vi "Decrypt Play Action.vi"(1 "Encrypted Play Action":string, 2 "Opponent's Move":T1) -> (0 "My Move":T1)   [LabVIEW 2020, in "AoC 2022.lvlib"]
uses:
  AoC 2022.lvlib
  Play Item.ctl
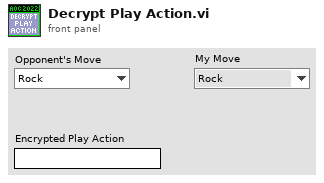
[diagram p1: front panel]
types:
  T1 = typedef "AoC 2022.lvlib/Play Item.ctl" = enum16{"Rock", "Paper", "Scissor"}
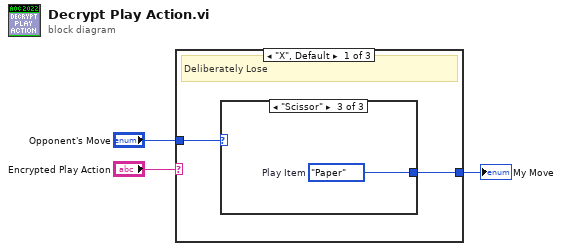
[diagram p0: block diagram]
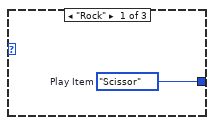
[diagram p2: hidden frame]
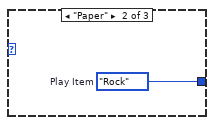
[diagram p3: hidden frame]
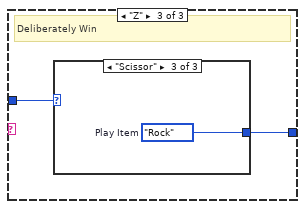
[diagram p5: hidden frame]
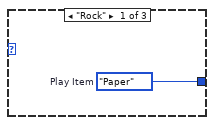
[diagram p6: hidden frame]
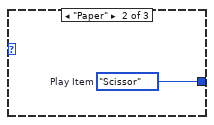
[diagram p7: hidden frame]
diagram:
  n1 = case shown="\"X\", Default" "Encrypted Play Action" {
    tunnel: [w5 w9 w11] -> w3
    tunnel: "Opponent's Move" -> [w4 w9 w10]
    frame "X", Default {
      # "Deliberately Lose"
      n2 = case shown="\"Scissor\"" w4 {
        tunnel: [w6 w7 w8] -> w5
        frame "Rock" {
          w6 = Play_Item."Scissor"  # Play Item
        }
        frame "Paper" {
          w7 = Play_Item."Rock"  # Play Item
        }
        frame "Scissor" {
          w8 = Play_Item."Paper"  # Play Item
        }
      }
    }
    frame "Y" {
      # "Deliberately Draw"
    }
    frame "Z" {
      # "Deliberately Win"
      n3 = case shown="\"Scissor\"" w10 {
        tunnel: [w12 w13 w14] -> w11
        frame "Rock" {
          w12 = Play_Item."Paper"  # Play Item
        }
        frame "Paper" {
          w13 = Play_Item."Scissor"  # Play Item
        }
        frame "Scissor" {
          w14 = Play_Item."Rock"  # Play Item
        }
      }
    }
  }
  "My Move" <- w3
